vi "Comparison - AC Temperature Control.vi"() -> ()   [LabVIEW 2016]
panel:
  out "Boolean":bool
  in  "Numeric":dbl
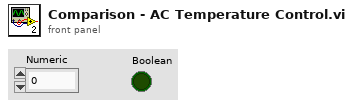
[diagram p1: front panel]
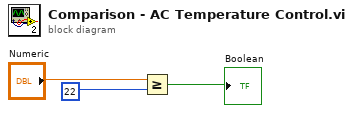
[diagram p0: block diagram]
diagram:
  n1 = Greater Or Equal?(x="Numeric", y=22) -> (x >= y?=→"Boolean":bool)
